vi "Control Path.vi"(11 "ImageButtonEditorPanel in":refnum<class "ImageButtonEditorPanel.lvclass">) -> (2 "Control Paths":path[](array[path]))   [LabVIEW 2020, in "VolatusGUIControls.lvlib" / "ImageButtonEditorPanel.lvclass"]
uses:
  ImageButtonEditorPanel.lvclass
  ImageButtonEditorPanel.lvclass/ImageButtonEditorPanel.ctl
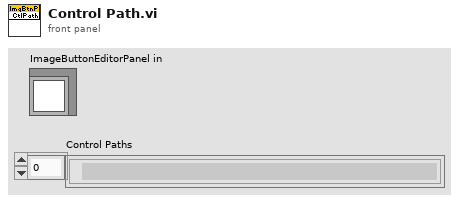
[diagram p1: front panel]
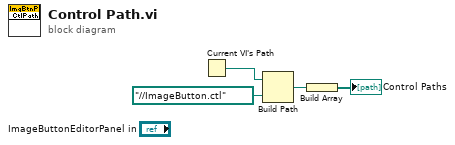
[diagram p0: block diagram]
diagram:
  n1 = Current VI's Path() -> (path=w4:path)
  n2 = Build Path(base path=w4, name or relative path=path "../../ImageButton.ctl") -> (appended path=w2:path)
  n3 = Build Array(w2) -> (→"Control Paths":path[])
